vi "SetValueByArrayName.vi"(0 "VI Reference In":refnum<vi>, 2 "delimiter (>>)":string=">>", 5 "Control Path":string, 7 "Name Array":T1[](array[typedef]), 11 "Error In":errorcluster) -> (4 "VI Reference Out":refnum<vi>, 15 "Error Out":errorcluster)   [LabVIEW 2016, in "Drona.lvlib" / "ControlValue.lvlib" / "StimulusListbox.lvlib"]
doc: "Sets value(signaling) for the multi select listbox control whose item names with its occurrence are specified. Set the value as 1 in occurrence to select the first occurrence of an item. \n\nThe input control name is given as a string , incase of path, use delimiters inbetween the path."
uses:
  StimulusListbox.lvlib
  typedef/Name&Occurrence.ctl
  <userlib>/_OpenG.lib/array/array.llb/Search 1D Array (String)__ogtk.vi
  <vilib>/Utility/error.llb/Error Cluster From Error Code.vi
  <vilib>/ErrorRing/Error Ring.xnode
  Drona.lvlib
  Get/GetControlRef/GetControlRef.lvlib
  ControlValue.lvlib
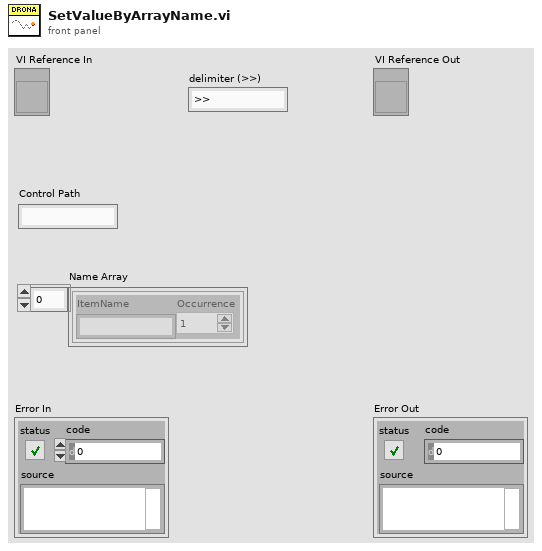
[diagram p1: front panel]
types:
  T1 = typedef "Drona.lvlib/ControlValue.lvlib/Name&Occurrence.ctl" = cluster{"ItemName":string, "Occurrence":i32}
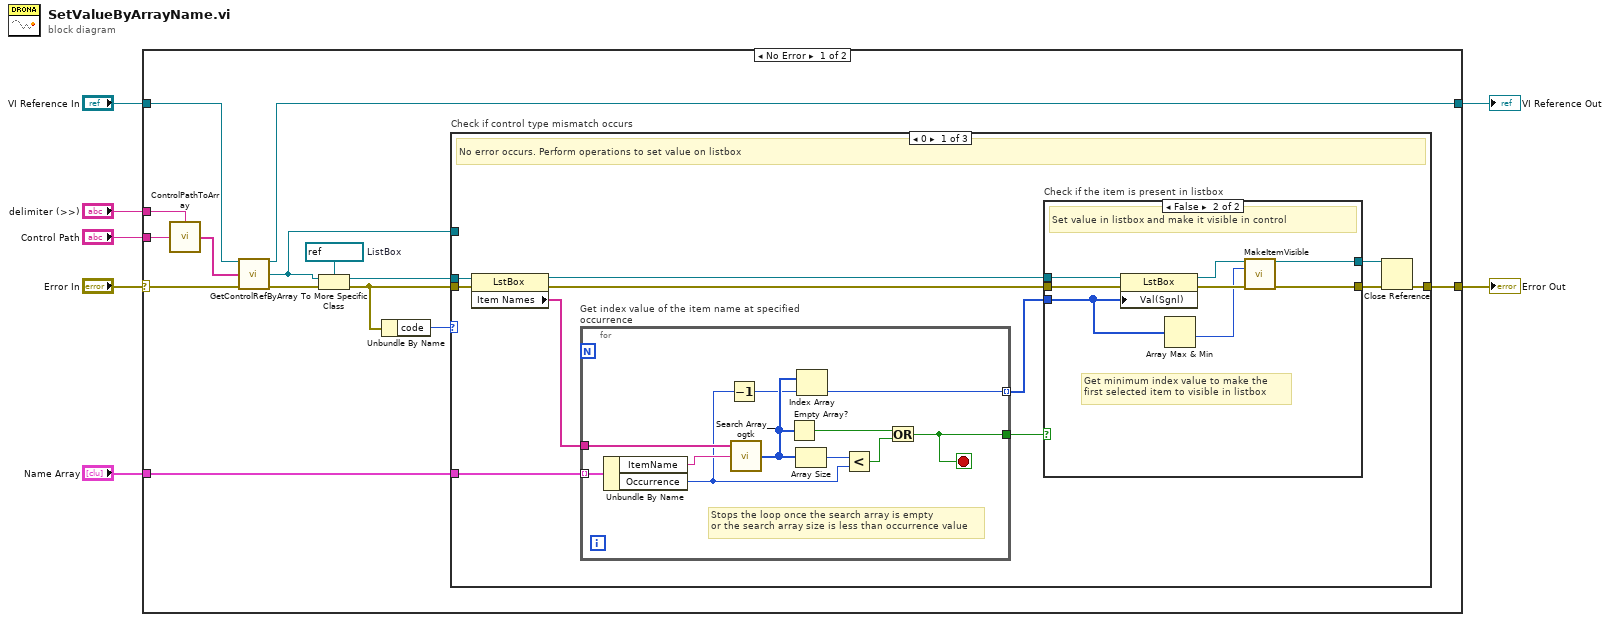
[diagram p0: block diagram]
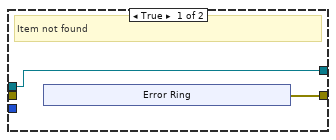
[diagram p2: hidden frame]
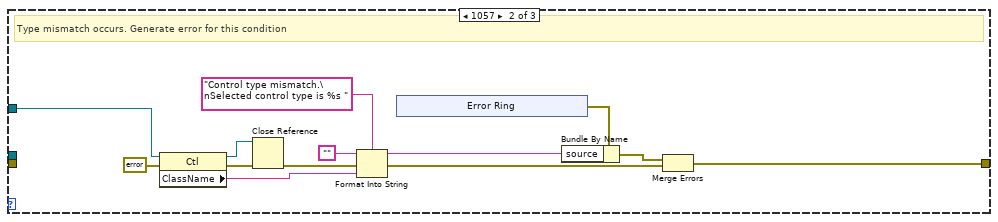
[diagram p3: hidden frame]
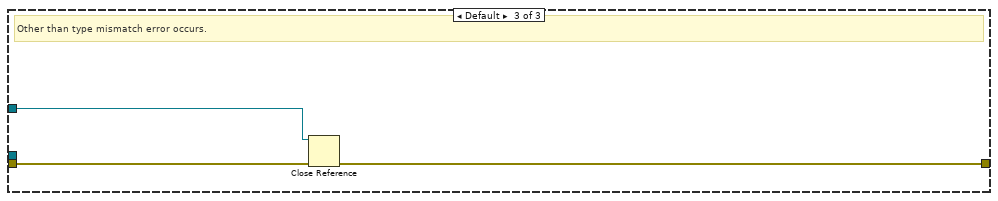
[diagram p4: hidden frame]
diagram:
  n1 = case shown="No Error" "Error In" {
    selector: "Error In" -> [w16 w81]
    tunnel: [w17 w81] -> w6
    tunnel: "VI Reference In" -> [w15 w80]
    tunnel: "Control Path" -> [w19 _]
    tunnel: [w12 w80] -> w3
    tunnel: "delimiter (>>)" -> [w18 _]
    tunnel: "Name Array" -> [w11 _]
    frame No Error {
      w21 = refnum<vi> refnum  # ListBox
      n2 = call "ControlPathToArray.vi"("Control Name"=w19, "delimiter (>>)"=w18) -> ("Control Path"=w14:string[])
      n3 = call "GetControlRefByArray.vi"("VI Reference In"=w15, "Control Path"=w14, "error In"=w16) -> ("VI Reference Out"=w12:refnum<vi>, "Ctl Refnum"=w8:refnum<vi>, "error out"=w13:errorcluster)  [unwired: 10 in]
      n4 = To More Specific Class(target class=w21, reference=w8, error in=w13) -> (specific class reference=w20:refnum<vi>, error out=w10:errorcluster)
      n5 = Unbundle By Name(w10) -> ("code"=w9:i32)
      n6 = case "Check if control type mismatch occurs" shown="0" w9 {
        tunnel: w10 -> [w32 _ w79]
        tunnel: w20 -> [w31 _ _]
        tunnel: [w30 w59 w78] -> w17
        tunnel: w11 -> [w26 _ _]
        tunnel: w8 -> [_ w60 w77]
        frame 0 {
          # "No error occurs. Perform operations to set value on listbox"
          n7 = property class="LstBox"(reference=w31, error in=w32) -> (reference out=w24:refnum<vi>, error out=w25:errorcluster, "Item Names"=w29:string[])
          n8 = for "Get index value of the item name at specified occurrence" {
            tunnel: w29 -> [w42]
            tunnel: w26 -> [w43] mode=indexing
            tunnel: [w34] -> w23 mode=indexing
            tunnel: [w33] -> w22
            stop <- w33 stop-if-true
            # "Stops the loop once the search array is empty \nor the search array size is less than occurrence value"
            n9 = Unbundle By Name(w43) -> ("ItemName"=w41:string, "Occurrence"=w36:i32)
            n10 = Decrement(x=w36) -> (x-1=w35:i32)
            n11 = call-poly <userlib>:"Search Array__ogtk.vi"("Array"=w42, "Element Data"=w41) -> ("Indices of Elements"=w37:i32[])  [unwired: 7 in]
            n12 = Empty Array?(array=w37) -> (empty?=w38:bool)
            n13 = Array Size(array=w37) -> (size(s)=w40:i32)
            n14 = Index Array(array=w37, index=w35) -> (element=w34:i32)
            n15 = Less?(x=w40, y=w36) -> (x < y?=w39:bool)
            n16 = Or(x=w38, y=w39) -> (x .or. y?=w33:bool)
          }
          n17 = case "Check if the item is present in listbox" shown="False" w22 {
            tunnel: [w45 w57] -> w28
            tunnel: [w44 w55] -> w27
            tunnel: w25 -> [_ w53]
            tunnel: w24 -> [w44 w52]
            tunnel: w23 -> [_ w51]
            frame True {
              # "Item not found"
              n18 = xnode "Error Ring"() -> ("error out"=w45:errorcluster)
            }
            frame False {
              # "Get minimum index value to make the \nfirst selected item to visible in listbox"
              # "Set value in listbox and make it visible in control"
              n19 = property class="LstBox"(reference=w52, error in=w53, "Val(Sgnl)"=w51) -> (reference out=w56:refnum<vi>, error out=w58:errorcluster)
              n20 = Array Max & Min(array=w51) -> (min value=w54:i32)  [unwired: 3 out]
              n21 = call "MakeItemVisible.vi"("ListBox Ref In"=w56, "Item Index"=w54, "Error In"=w58) -> ("ListBox Ref Out"=w55:refnum<vi>, "Error Out"=w57:errorcluster)  [unwired: 11 in]
            }
          }
          n22 = Close Reference(reference=w27, error in (no error)=w28) -> (error out=w30:errorcluster)
        }
        frame 1057 {
          # "Type mismatch occurs. Generate error for this condition"
          n23 = property class="Ctl"(reference=w60, error in=errorcluster {"status"=FALSE, "code"=0, "source"=""} ("error out")) -> (reference out=w61:refnum<vi>, error out=w71:errorcluster, "ClassName"=w68:string)
          n24 = Close Reference(reference=w61, error in (no error)=w71) -> (error out=w62:errorcluster)
          n25 = Format Into String(format string="Control type mismatch.\nSelected control type is %s ", initial string="", error in=w62, w68) -> (resulting string=w65:string, error out=w63:errorcluster)
          n26 = xnode "Error Ring"() -> ("error out"=w66:errorcluster)
          n27 = Bundle By Name(cluster=w66, "source"=w65) -> (w64:errorcluster)
          n28 = Merge Errors(w64, w63) -> (w59:errorcluster)
        }
        frame Default {
          # "Other than type mismatch error occurs."
          n29 = Close Reference(reference=w77, error in (no error)=w79) -> (error out=w78:errorcluster)
        }
      }
    }
    frame Error {
    }
  }
  "Error Out" <- w6
  "VI Reference Out" <- w3
